vi "closeApps.vi"(8 "error in (no error)":errorcluster, 11 "CameraManager in":refnum<class "CameraManager.lvclass">) -> (0 "error out":errorcluster, 3 "CameraManager out":refnum<class "CameraManager.lvclass">)   [LabVIEW 2009, in "iManagement.lvlib" / "CameraManager.lvclass"]
doc: "Close down the camera"
uses:
  CameraManager.lvclass
  CameraManager.lvclass/CameraManager.ctl
  Hal/Channels/Camera/CameraController.lvclass
  Hal/Channels/Camera/CameraEventsManager/CameraEventsManger.lvclass
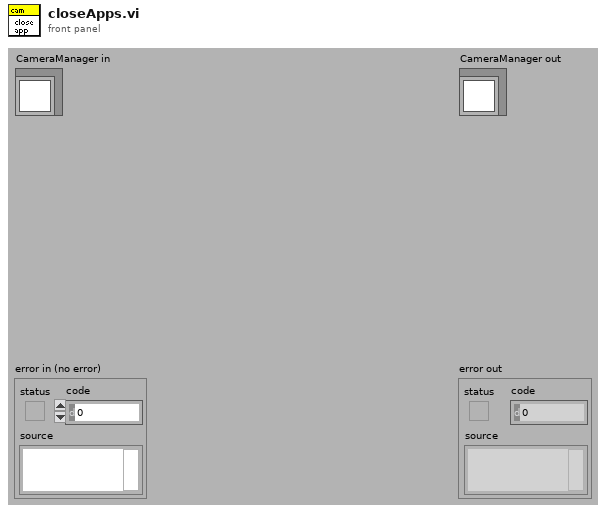
[diagram p1: front panel]
types:
  T1 = cluster{"settingsFrontEndEvents":cluster{"loadSettingsFromPath":refnum<user-event>, "lookUpElementEvent":refnum<user-event>, "saveSettings":refnum<user-event>, "loadSettings":refnum<user-event>, "close":refnum<user-event>, "replaceElement":refnum<user-event>, "findParentNodes":refnum<user-event>, "createNode":refnum<user-event>}, "settingBackEndEvents":cluster{"defaultSettingsPathRequest":refnum<user-event>, "searchResultEvent":refnum<user-event>, "settingsSaved":refnum<user-event>, "settingsLoaded":refnum<user-event>, "foundParentNode":refnum<user-event>}}
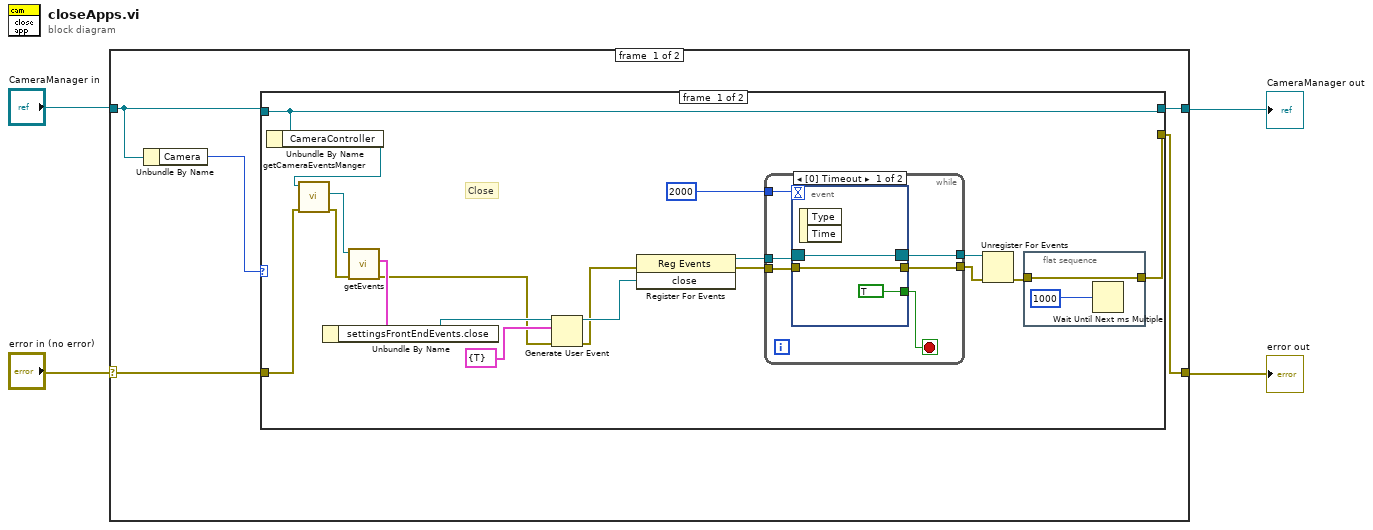
[diagram p0: block diagram]
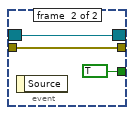
[diagram p2: hidden frame]
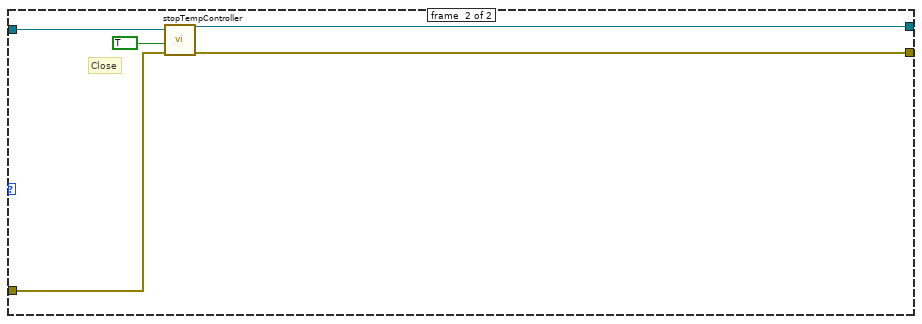
[diagram p3: hidden frame]
diagram:
  n1 = case shown="No Error" "error in (no error)" {
    selector: "error in (no error)" -> [w9 w48]
    tunnel: [w6 w48] -> w3
    tunnel: [w5 w47] -> w1
    tunnel: "CameraManager in" -> [w7 w47]
    frame #0 {
      n2 = Unbundle By Name(w7) -> ("Camera"=w8:enum16{"AndorIKon", "ICCamera"})
      n3 = case shown="\"ICCamera\", Default" w8 {
        tunnel: w9 -> [w26 w44]
        tunnel: w7 -> [w13 w46]
        tunnel: [w12 w43] -> w6
        tunnel: [w13 w42] -> w5
        frame #0 {
          # "Close"
          n4 = Unbundle By Name(w13) -> ("CameraController"=w11:refnum<class "CameraController.lvclass">)
          n5 = call-dynamic "getCameraEventsManger.vi"("error in (no error)"=w26, "CameraController.lvclass in"=w11) -> ("error out"=w17:errorcluster, "Hardware:Channels.lvlib:CameraEventsManger.lvclass"=w18:refnum<class "CameraEventsManger.lvclass">)  [unwired: 7 in, 1 out]
          n6 = call-dynamic "getEvents.vi"("error in (no error)"=w17, "CameraEventsManger in"=w18) -> ("error out"=w15:errorcluster, "settingsEvents"=w16:T1)  [unwired: 5 in, 3 out]
          n7 = Unbundle By Name(w16) -> ("settingsFrontEndEvents.close"=w19:refnum<user-event>)
          n8 = Generate User Event(user event=w19, event data cluster=cluster{"dummy":bool} {"dummy"=TRUE} ("event data"), error in=w15) -> (user event out=w25:refnum<user-event>, error out=w22:errorcluster)
          n9 = register-events(error in=w22, w25) -> (reference out=w24:refnum<event-registration>, error out=w23:errorcluster)  [unwired: 1 in]
          n10 = while {
            tunnel: w24 -> [w35]
            tunnel: w23 -> [w34]
            tunnel: [w33] -> w20
            tunnel: [w32] -> w21
            tunnel: 2000 -> [w30]
            stop <- w31 stop-if-true
            n11 = event shown="[0] Timeout" {
              selector: w35 -> [w38 w41]
              dyn-events: [w38 w41] -> w32
              timeout: w30 -> [_ _]
              tunnel: w34 -> [w37 w40]
              tunnel: [w37 w40] -> w33
              tunnel: [TRUE TRUE] -> w31
              event #0 {
                n12 = event-data() -> ()  [unwired: 1 in, 2 out]
              }
              event #1 {
                n13 = event-data() -> ()  [unwired: 1 in, 1 out]
              }
            }
          }
          n14 = Unregister For Events(event registration refnum=w21, error in=w20) -> (error out=w14:errorcluster)
          n15 = flat-sequence {
            tunnel: w14 -> [w29]
            tunnel: [w29] -> w12
            frame #0 {
              n16 = Wait Until Next ms Multiple(millisecond multiple=1000) -> ()  [unwired: 1 out]
            }
          }
        }
        frame #1 {
          # "Close"
          n17 = call "stopTempController.vi"("error in (no error)"=w44, "releaseWhenReady"=TRUE, "CameraManager in"=w46) -> ("error out"=w43:errorcluster, "CameraManager out"=w42:refnum<class "CameraManager.lvclass">)  [unwired: 7 in]
        }
      }
    }
    frame #1 {
    }
  }
  "error out" <- w3
  "CameraManager out" <- w1
